vi "练习-y=kx+b.vi"() -> ()   [LabVIEW 2013]
panel:
  out "波形图表":dbl(graph)
  out "y=kx+b":dbl
  in  "b":dbl
  in  "k":dbl
  in  "停止":bool
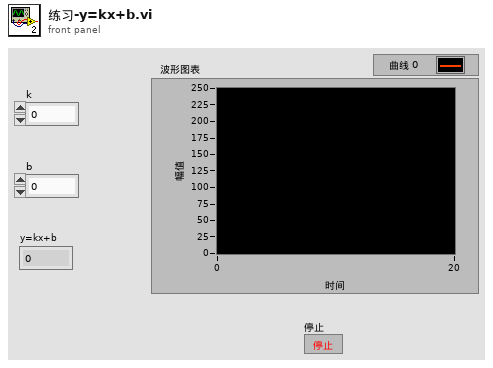
[diagram p1: front panel]
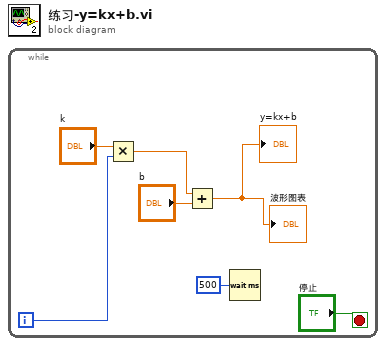
[diagram p0: block diagram]
diagram:
  n1 = while {
    i -> [w5]
    stop <- "停止" stop-if-true
    n2 = Multiply(x="k", y=w5) -> (x*y=w4:dbl)
    n3 = Add(x=w4, y="b") -> (x+y=→"y=kx+b" →"波形图表":dbl)
    n4 = Wait (ms)(milliseconds to wait=u32 500 ("等待时间（毫秒）")) -> ()  [unwired: 1 out]
  }
